vi "Stop Acquisition.vi"(8 "error in (no error)":errorcluster, 11 "Hardware Resources in":T1={"VISA resource name"="", "DAQ Type"=0, "Channel 1"={"Acquiring"=FALSE, "Enabled"=FALSE, "Terminal configuration"=32767, "Range"=0, "Coupling"=0}, "Channel 2"={"Acquiring"=FALSE, "Enabled"=FALSE, "Terminal configuration"=0, "Range"=0, "Coupling"=0}, "Timing"={"Sample Time [Time Units]"=0, "Actual Sample Time [s]"=0.0, "Samples per Iteration"=0, "Sample Clock Source"=0, "Time Units"=0, "t0"=timestamp(0 s since 1904-01-01), "Baud rate"=0}, "PS Parameters"={"PS handle"=0, "PS Max_adc"=32767, "PS Enabled Array"=[], "PS Device Info"={"Driver Version"="", "USB Version"="", "Hardware"="", "Variant"="", "Batch and Serial"="", "Cal Date"="", "Kernel Version"="", "Digital HW Version"="", "Analogue HW Version"="", "Firmware 1"="", "Firmware 2"="", "MSO"=FALSE, "Number of Channels"=0}, "Channel 1 Buffer"=refnum, "Channel 2 Buffer"=refnum, "Resolution"=0, "USB Power"=FALSE}, "Trigger"={"Direction"=0, "Threshold [V]"=0.0, "Enabled"=FALSE, "Trigger Source"=0}, "Keithley Parameters"={"Previous End / Current Start"=0, "Quantity"=0}} {"Keithley Parameters"."Quantity" items=["Current", "Voltage"]; "Trigger"."Trigger Source" items=["Channel 1"=0, "Channel 2"=1, "Ext."=4]; "Trigger"."Direction" items=["Falling", "Rising"]; "PS Parameters"."Resolution" items=["8", "12", "14", "15", "16"]; "Timing"."Time Units" items=["Seconds"]; "Timing"."Sample Clock Source" items=["Internal", "External"]; "Channel 2"."Coupling" items=["AC", "DC"]; "Channel 2"."Range" items=["0.01", "0.02", "0.05", "0.1", "0.2", "0.5", "1", "2", "5", "10", "20", "50", "100", "1000"]; "Channel 2"."Terminal configuration" items=["Referenced Single Ended", "Differential"]; "Channel 1"."Coupling" items=["AC", "DC"]; "Channel 1"."Range" items=["0.01", "0.02", "0.05", "0.1", "0.2", "0.5", "1", "2", "5", "10", "20", "50", "100", "1000"]; "Channel 1"."Terminal configuration" items=["Referenced Single Ended", "Differential"]; "DAQ Type" items=["Simulated", "Tektronics DPO2k/3k/4k", "PicoScope 2000a Series", "Keithley DMM7510", "PicoScope 5000a Series", "Arduino"]}) -> (0 "error out":errorcluster)   [LabVIEW 2017, in "Acquisition.lvlib"]
doc: "Stops the acquisition."
uses:
  Acquisition.lvlib
  Hardware Configuration.ctl
  Signal Type.ctl
  Settings/Terminal Configuration.ctl
  Settings/Range.ctl
  Settings/Coupling.ctl
  Settings/Sampling Clock Source.ctl
  Settings/Time Units.ctl
  Settings/Resolution.ctl
  Settings/Trigger Direction.ctl
  Settings/Trigger Source.ctl
  Settings/Quantity.ctl
  support/DAQ Drivers/Tektronix DPO MSO 2000 4000 Series/Tektronix DPO MSO 2000 4000 Series.lvlib
  support/DAQ Drivers/Keithley DMM7510/Keithley DMM7510.lvlib
  C:/RPF_dlls/PS5000a/ps5000a.dll
  Settings/Settings.lvlib
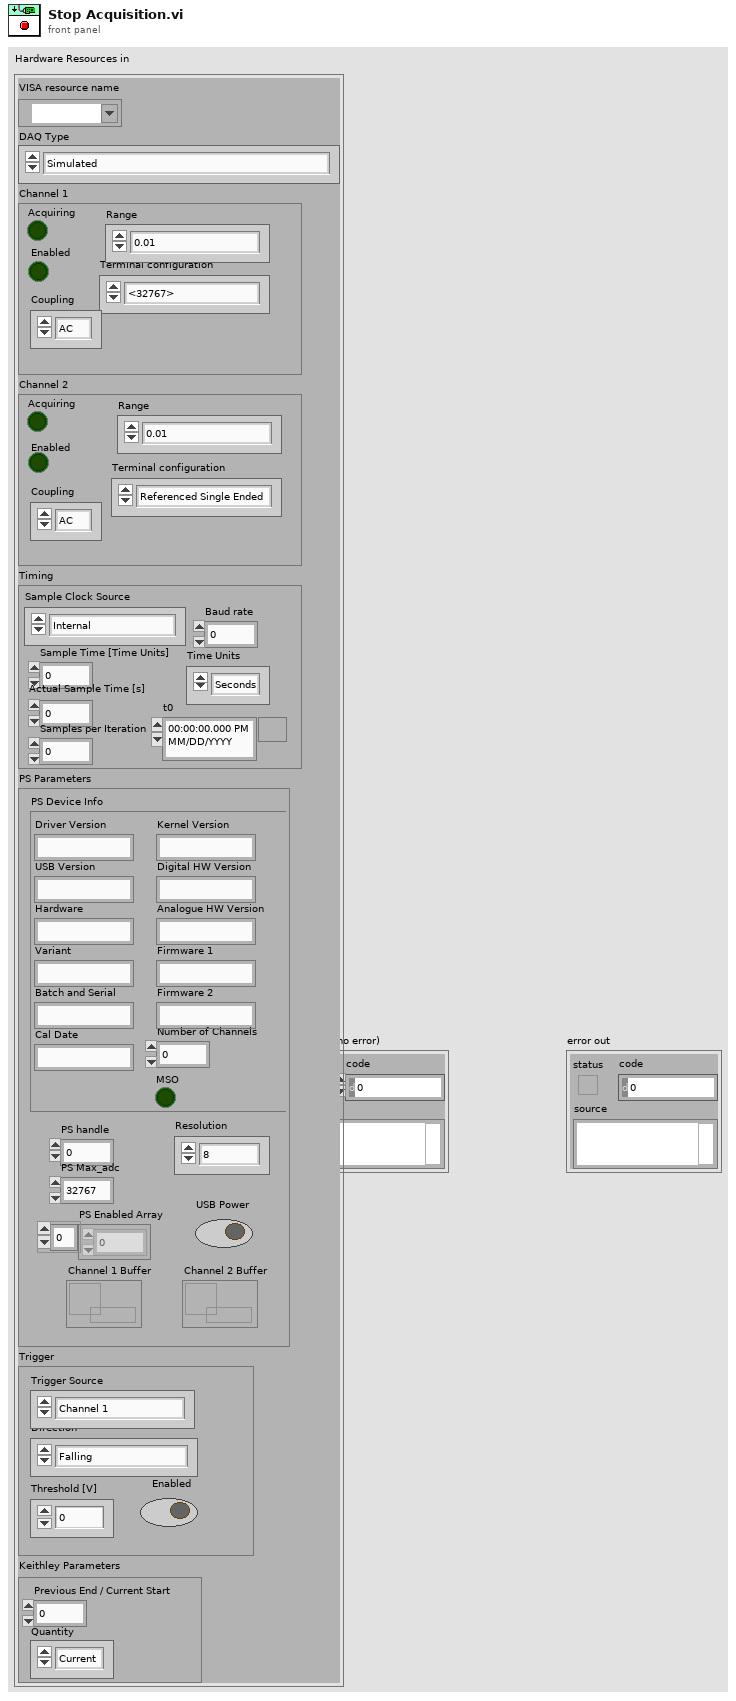
[diagram p1: front panel]
types:
  T1 = typedef "Acquisition.lvlib/Hardware Configuration.ctl" = cluster{"VISA resource name":refnum<visa-resource-name>, "DAQ Type":T2, "Channel 1":cluster{"Acquiring":bool, "Enabled":bool, "Terminal configuration":T3, "Range":T4, "Coupling":T5}, "Channel 2":cluster{"Acquiring":bool, "Enabled":bool, "Terminal configuration":T3, "Range":T4, "Coupling":T5}, "Timing":cluster{"Sample Time [Time Units]":u32, "Actual Sample Time [s]":dbl, "Samples per Iteration":u32, "Sample Clock Source":T6, "Time Units":T7, "t0":timestamp, "Baud rate":u32}, "PS Parameters":cluster{"PS handle":i16, "PS Max_adc":i16, "PS Enabled Array":i16[], "PS Device Info":cluster{"Driver Version":string, "USB Version":string, "Hardware":string, "Variant":string, "Batch and Serial":string, "Cal Date":string, "Kernel Version":string, "Digital HW Version":string, "Analogue HW Version":string, "Firmware 1":string, "Firmware 2":string, "MSO":bool, "Number of Channels":i16}, "Channel 1 Buffer":refnum<data-value>, "Channel 2 Buffer":refnum<data-value>, "Resolution":T8, "USB Power":bool}, "Trigger":cluster{"Direction":T9, "Threshold [V]":dbl, "Enabled":bool, "Trigger Source":T10}, "Keithley Parameters":cluster{"Previous End / Current Start":i32, "Quantity":T11}}
  T2 = typedef "Acquisition.lvlib/Signal Type.ctl" = u16
  T3 = typedef "Settings.lvlib/Terminal Configuration.ctl" = u16
  T4 = typedef "Settings.lvlib/Range.ctl" = u16
  T5 = typedef "Settings.lvlib/Coupling.ctl" = i16
  T6 = typedef "Settings.lvlib/Sampling Clock Source.ctl" = u16
  T7 = typedef "Settings.lvlib/Time Units.ctl" = u32
  T8 = typedef "Settings.lvlib/Resolution.ctl" = i32
  T9 = typedef "Settings.lvlib/Trigger Direction.ctl" = u16
  T10 = typedef "Settings.lvlib/Trigger Source.ctl" = u16
  T11 = typedef "Settings.lvlib/Quantity.ctl" = u16
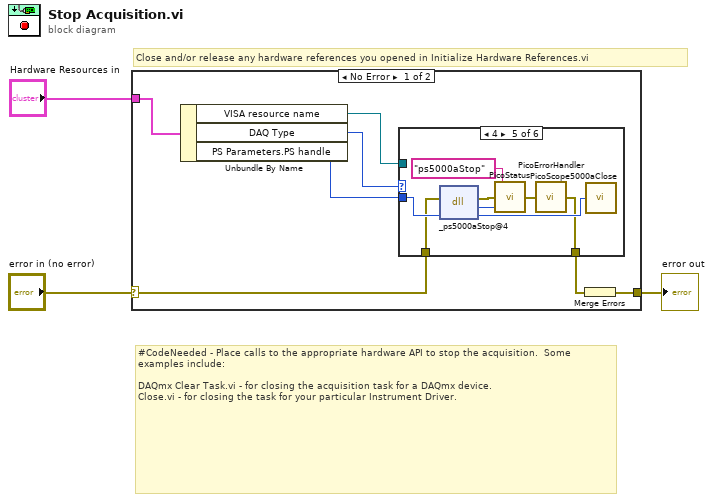
[diagram p0: block diagram]
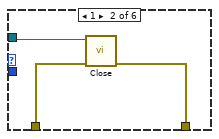
[diagram p3: hidden frame]
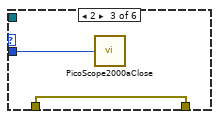
[diagram p4: hidden frame]
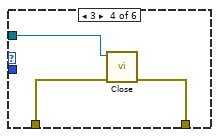
[diagram p5: hidden frame]
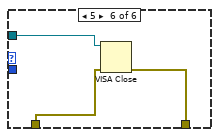
[diagram p6: hidden frame]
diagram:
  # "#CodeNeeded - Place calls to the appropriate hardware API to stop the acquisition.  Some examples include:\n\nDAQmx Clear Task.vi - for closing the acquisition task for a DAQmx device.\nClose.vi - for closing the task for your particular Instrument Driver."
  # "Close and/or release any hardware references you opened in Initialize Hardware References.vi"
  n1 = case shown="No Error" "error in (no error)" {
    selector: "error in (no error)" -> [w7 w31]
    tunnel: [w10 w31] -> w2
    tunnel: "Hardware Resources in" -> [w9 _]
    frame No Error {
      n2 = Unbundle By Name(w9) -> ("VISA resource name"=w8:refnum<visa-resource-name>, "DAQ Type"=w5:T2, "PS Parameters.PS handle"=w4:i16)
      n3 = case shown="4" w5 {
        tunnel: w8 -> [_ w14 _ w19 _ w30]
        tunnel: w7 -> [w11 w13 w15 w18 w26 w29]
        tunnel: [w11 w12 w15 w17 w20 w28] -> w6
        tunnel: w4 -> [_ _ w16 _ w27 _]
        frame 0, Default {
        }
        frame 1 {
          n4 = call "Close.vi"("error in (no error)"=w13, "VISA resource name"=w14) -> ("error out"=w12:errorcluster)  [unwired: 9 in]
        }
        frame 2 {
          n5 = call "PicoScope2000aClose.vi"("handle"=w16) -> ()
        }
        frame 3 {
          n6 = call "Close.vi"("error in (no error)"=w18, "VISA resource name"=w19) -> ("error out"=w17:errorcluster)  [unwired: 9 in]
        }
        frame 4 {
          n7 = dll-call lib="C:/RPF_dlls/PS5000a/ps5000a.dll" fn="_ps5000aStop@4"(error in=w26, "handle"=w27) -> (error out=w24:errorcluster, "PICO_STATUS"=w23:u32, "handle"=w21:i16)  [unwired: 2 in, 1 out]
          n8 = call "PicoStatus.vi"("PICO STATUS"=w23, "error in"=w24, "source"="ps5000aStop") -> ("error out"=w22:errorcluster)
          n9 = call "PicoErrorHandler.vi"("error in"=w22) -> ("error out"=w20:errorcluster)
          n10 = call "PicoScope5000aClose.vi"("handle"=w21) -> ()
        }
        frame 5 {
          n11 = VISA Close(VISA resource name=w30, error in (no error)=w29) -> (error out=w28:errorcluster)
        }
      }
      n12 = Merge Errors(w6) -> (w10:errorcluster)
    }
    frame Error {
    }
  }
  "error out" <- w2
